vi "AlliGator MCP Voltage to Gain.vi"(9 "MCP Parameters":T1={"G0"=3.0, "A"=4.052e-06, "V0"=174.3, "B"=0.0422, "g"=0.322}, 11 "MCP Voltage":dbl) -> (3 "Gain":dbl)   [LabVIEW 2021, in "AlliGator Intensity Corrections.lvlib"]
doc: "Heuristic fit of the relationship between effective ICCD gain G and MCP voltage V_MCP.\n\nThe function used is a stretched exponential with vertical and horizontal offsets.\n\nParameters need to be fitted independetly with a G(V_MCP) series."
uses:
  AlliGator Intensity Corrections.lvlib
panel:
  # "see the AlliGator License on the block diagram (Ctrl+E or Window:Show Block Diagram)"
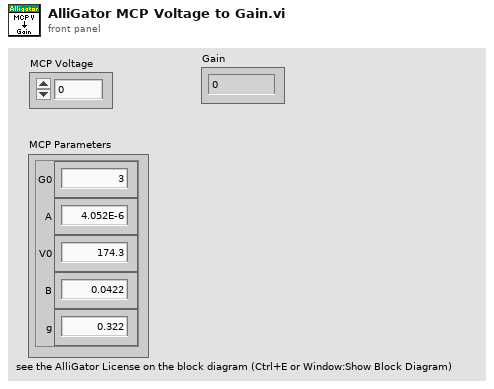
[diagram p1: front panel]
types:
  T1 = cluster{"G0":dbl, "A":dbl, "V0":dbl, "B":dbl, "g":dbl}
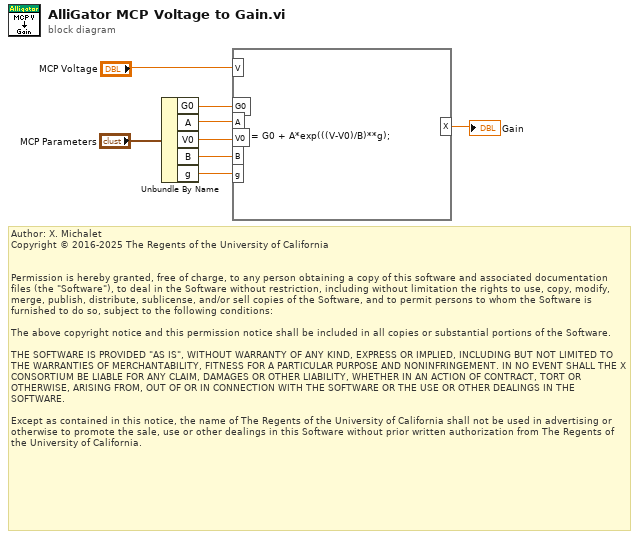
[diagram p0: block diagram]
diagram:
  # "Author: X. Michalet\nCopyright © 2016-2025 The Regents of the University of California\n \n\nPermission is hereby granted, free of charge, to any person obtaining a copy of this software and associated documentation files (the \"Software\"), to deal in the Software without restriction, including without limitation the rights to use, copy, modify, merge, publish, distribute, sublicense, and/or sell copies of the Software, and to permit persons to whom the Software is furnished to do so, subject to the following conditions:\n\nThe above copyright notice and this permission notice shall be included in all copies or substantial portions of the Software.\n\nTHE SOFTWARE IS PROVIDED \"AS IS\", WITHOUT WARRANTY OF ANY KIND, EXPRESS OR IMPLIED, INCLUDING BUT NOT LIMITED TO THE WARRANTIES OF MERCHANTABILITY, FITNESS FOR A PARTICULAR PURPOSE AND NONINFRINGEMENT. IN NO EVENT SHALL THE X CONSORTIUM BE LIABLE FOR ANY CLAIM, DAMAGES OR OTHER LIABILITY, WHETHER IN AN ACTION OF CONTRACT, TORT OR OTHERWISE, ARISING FROM, OUT OF OR IN CONNECTION WITH THE SOFTWARE OR THE USE OR OTHER DEALINGS IN THE SOFTWARE.\n\nExcept as contained in this notice, the name of The Regents of the University of California shall not be used in advertising or otherwise to promote the sale, use or other dealings in this Software without prior written authorization from The Regents of the University of California."
  n1 = Unbundle By Name("MCP Parameters") -> ("G0"=w5:dbl, "A"=w4:dbl, "V0"=w3:dbl, "B"=w2:dbl, "g"=w1:dbl)
  n2 = formula code="X = G0 + A*exp(((V-V0)/B)**g);"("V"="MCP Voltage", "G0"=w5, "A"=w4, "V0"=w3, "B"=w2, "g"=w1) -> ("X"=→"Gain":dbl)
